vi "Serial Comunication.vi"(6 "parity (0:none)":enum16{"None", "Odd", "Even", "Mark", "Space"}(ring)=enum."Odd", 8 "error in (no error)":errorcluster, 9 "write buffer":string, 10 "baud rate (9600)":u32=115200, 11 "VISA resource name":refnum<visa-resource-name>) -> (0 "error out":errorcluster, 2 "Result":string, 3 "VISA resource name out":refnum<visa-resource-name>)   [LabVIEW 2020]
uses:
  f80ddd37-9d09-4cc6-bb77-6b2823155c5b.vi
  <vilib>/Instr/_visa.llb/VISA Configure Serial Port (Instr).vi
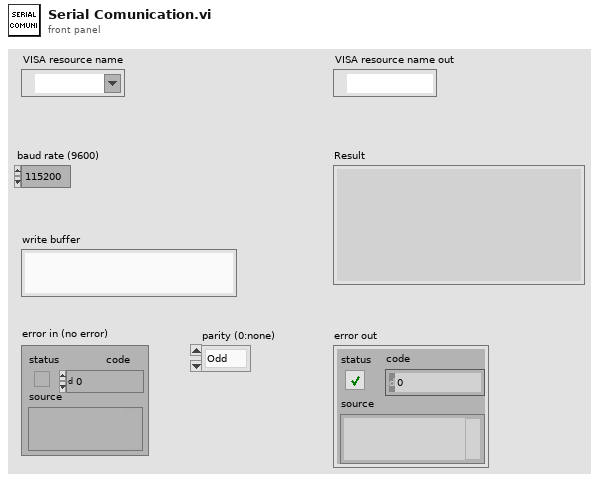
[diagram p1: front panel]
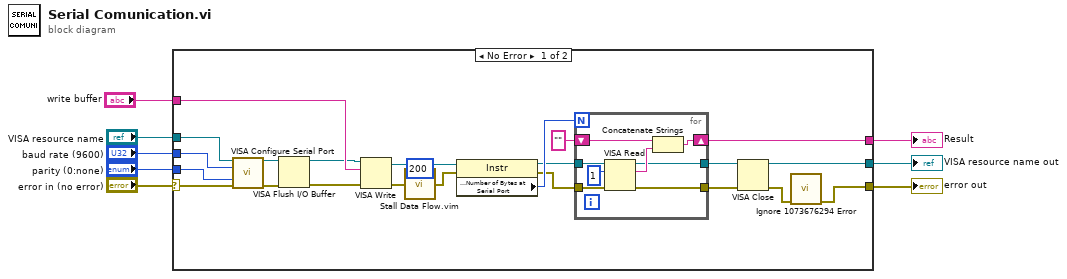
[diagram p0: block diagram]
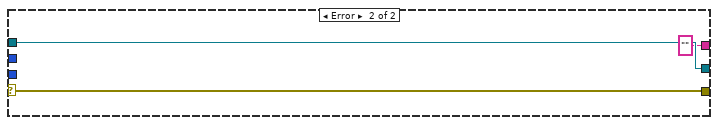
[diagram p2: hidden frame]
diagram:
  n1 = case shown="No Error" "error in (no error)" {
    selector: "error in (no error)" -> [w27 w41]
    tunnel: "VISA resource name" -> [w30 w40]
    tunnel: "baud rate (9600)" -> [w29 _]
    tunnel: "parity (0:none)" -> [w28 _]
    tunnel: "write buffer" -> [w26 _]
    tunnel: [w17 w40] -> w3
    tunnel: [w16 ""] -> w2
    tunnel: [w9 w41] -> w1
    frame No Error {
      n2 = call-poly "VISA Configure Serial Port"("VISA resource name"=w30, "baud rate (9600)"=w29, "parity (0:none)"=w28, "error in (no error)"=w27) -> ("VISA resource name out"=w13:refnum<visa-resource-name>, "error out"=w14:errorcluster)  [unwired: 10 in]
      n3 = VISA Flush I/O Buffer(VISA resource name=w13, error in (no error)=w14) -> (VISA resource name out=w11:refnum<visa-resource-name>, error out=w12:errorcluster)  [unwired: 1 in]
      n4 = VISA Write(VISA resource name=w11, write buffer=w26, error in (no error)=w12) -> (VISA resource name out=w22:refnum<visa-resource-name>, error out=w25:errorcluster)  [unwired: 1 out]
      n5 = call "Stall Data Flow.vim"("value in"=w25, "milliseconds to wait"=u32 200) -> ("value out"=w23:errorcluster)  [unwired: 1 out]
      n6 = property class="Instr"(reference=w22, error in=w23) -> (reference out=w19:refnum<visa-resource-name>, error out=w20:errorcluster, "Serial Settings:Number of Bytes at Serial Port"=w21:u32)
      n7 = for {
        N: w21 -> [_]
        tunnel: w20 -> [w38]
        tunnel: w19 -> [w37]
        shift-right: [w35] -> w16
        shift-left: "" -> [w34]
        tunnel: [w32] -> w18
        tunnel: [w31] -> w17
        n8 = VISA Read(VISA resource name=w37, byte count=u32 1, error in (no error)=w38) -> (VISA resource name out=w31:refnum<visa-resource-name>, read buffer=w33:string, error out=w32:errorcluster)  [unwired: 1 out]
        n9 = Concatenate Strings(w34, w33) -> (w35:string)
      }
      n10 = VISA Close(VISA resource name=w17, error in (no error)=w18) -> (error out=w10:errorcluster)
      n11 = call "Ignore 1073676294 Error.vi"("error in (no error)"=w10) -> ("error out"=w9:errorcluster)  [unwired: 10 in]
    }
    frame Error {
    }
  }
  "VISA resource name out" <- w3
  "error out" <- w1
  "Result" <- w2
